vi "Analog_16Ch_Datalogging.vi"() -> ()   [LabVIEW 2013]
uses:
  <vilib>/DAQmx/read.llb/DAQmx Read (Analog 1D Wfm NChan NSamp).vi
  <vilib>/DAQmx/create/channels.llb/DAQmx Create Channel (AI-Voltage-Basic).vi
  <vilib>/DAQmx/configure/timing.llb/DAQmx Timing (Sample Clock).vi
  <vilib>/DAQmx/miscellaneous.llb/DAQmx Fill In Error Info.vi
panel:
  in  "Filename":path=path "C:/Temp/test100614.lvm"
  in  "stop":bool
  in  "Start/Stop":bool
  in  "USB-6008":tag="Dev1/ai0"
  out "USB 6008":waveform(dbl)[](graph)
  out "USB 6009":waveform(dbl)[](graph)
  in  "USB-6009":tag="Dev1/ai0"
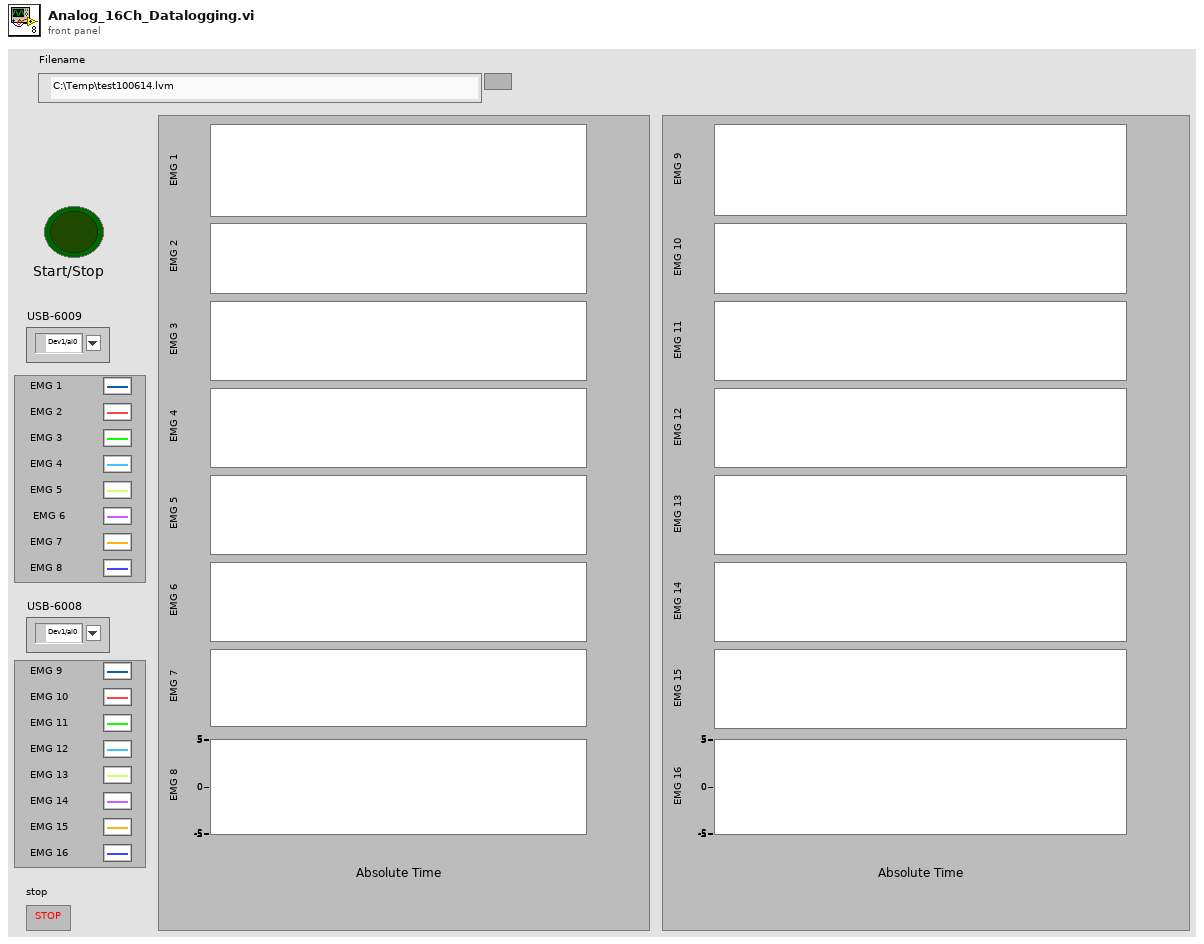
[diagram p1: front panel]
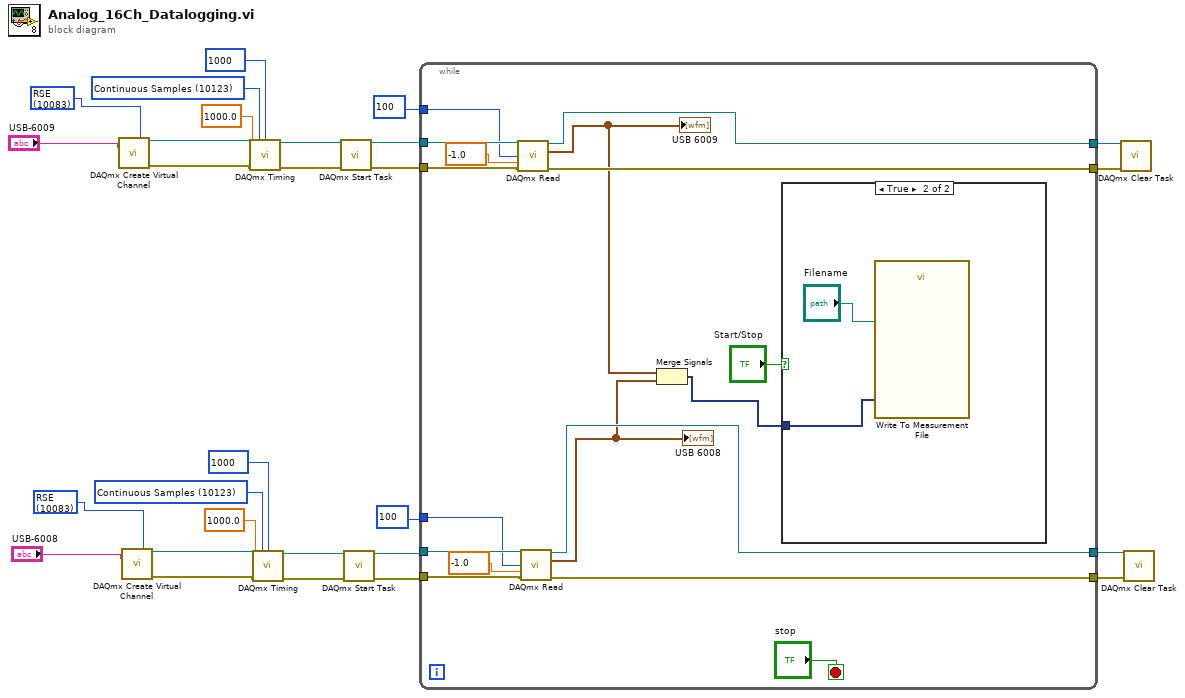
[diagram p0: block diagram]
diagram:
  w14 = 10083 items=["default"=-1, "RSE"=10083, "NRSE"=10078, "Differential"=10106, "Pseudodifferential"=12529] ("input terminal configuration")
  w12 = 10123 items=["Continuous Samples"=10178, "Continuous Samples"=10123, "Hardware Timed Single Point"=12522] ("sample mode")
  w15 = 10083 items=["default"=-1, "RSE"=10083, "NRSE"=10078, "Differential"=10106, "Pseudodifferential"=12529] ("input terminal configuration")
  w17 = 10123 items=["Continuous Samples"=10178, "Continuous Samples"=10123, "Hardware Timed Single Point"=12522] ("sample mode")
  n1 = call-poly <vilib>:"DAQmx Create Virtual Channel.vi"("input terminal configuration"=w15, "physical channels"="USB-6009") -> ("task out"=w28:refnum<k21>, "error out"=w27:errorcluster)  [unwired: 12 in]
  n2 = call-poly <vilib>:"DAQmx Create Virtual Channel.vi"("input terminal configuration"=w14, "physical channels"="USB-6008") -> ("task out"=w1:refnum<k21>, "error out"=w2:errorcluster)  [unwired: 12 in]
  n3 = call-poly <vilib>:"DAQmx Timing.vi"("task/channels in"=w28, "sample mode"=w17, "samples per channel"=1000, "rate"=1000.0, "error in"=w27) -> ("task out"=w26:refnum<k21>, "error out"=w25:errorcluster)  [unwired: 9 in]
  n4 = call-poly <vilib>:"DAQmx Timing.vi"("task/channels in"=w1, "sample mode"=w12, "samples per channel"=1000, "rate"=1000.0, "error in"=w2) -> ("task out"=w3:refnum<k21>, "error out"=w4:errorcluster)  [unwired: 9 in]
  n5 = call <vilib>:"DAQmx Start Task.vi"("task/channels in"=w26, "error in"=w25) -> ("task out"=w22:refnum<k21>, "error out"=w23:errorcluster)  [unwired: 12 in]
  n6 = call <vilib>:"DAQmx Start Task.vi"("task/channels in"=w3, "error in"=w4) -> ("task out"=w7:refnum<k21>, "error out"=w6:errorcluster)  [unwired: 12 in]
  n7 = while {
    tunnel: w23 -> [w45]
    tunnel: w22 -> [w44]
    tunnel: [w43] -> w21
    tunnel: [w42] -> w20
    tunnel: 100 ("number of samples per channel") -> [w41]
    tunnel: 100 ("number of samples per channel") -> [w29]
    tunnel: [w40] -> w9
    tunnel: [w39] -> w8
    tunnel: w7 -> [w38]
    tunnel: w6 -> [w37]
    stop <- "stop" stop-if-true
    n8 = call-poly <vilib>:"DAQmx Read.vi"("task/channels in"=w44, "number of samples per channel"=w41, "timeout"=-1.0, "error in"=w45) -> ("task out"=w43:refnum<k21>, "data"=w33:waveform(dbl)[], "error out"=w42:errorcluster)  [unwired: 9 in]
    "USB 6009" <- w33
    n9 = call-poly <vilib>:"DAQmx Read.vi"("task/channels in"=w38, "number of samples per channel"=w29, "timeout"=-1.0, "error in"=w37) -> ("task out"=w39:refnum<k21>, "data"=w34:waveform(dbl)[], "error out"=w40:errorcluster)  [unwired: 9 in]
    "USB 6008" <- w34
    n10 = Merge Signals(w33, w34) -> (w32:dynamicdata)
    n11 = case shown="True" "Start/Stop" {
      tunnel: w32 -> [_ w47]
      frame False {
      }
      frame True {
        n12 = call "Write To Measurement File"("Signals"=w47, "Filename"="Filename") -> ()  [unwired: 15 in, 3 out]
      }
    }
  }
  n13 = call <vilib>:"DAQmx Clear Task.vi"("task in"=w21, "error in"=w20) -> ()  [unwired: 13 in, 1 out]
  n14 = call <vilib>:"DAQmx Clear Task.vi"("task in"=w8, "error in"=w9) -> ()  [unwired: 13 in, 1 out]
